vi "test Get Faultable Parameter.vi"() -> ()   [LabVIEW 2023, in "Scripting.lvclass"]
uses:
  Scripting.lvclass
  Scripting.lvclass/Scripting.ctl
  <vilib>/NI/NI VeriStand Encoding and Decoding/Encoding.ctl
  <vilib>/NI/NI VeriStand Encoding and Decoding/Encoding and Decoding.lvlib
  Shared/Parameter Definition.ctl
  Shared/Direction.ctl
  Shared/SDI.ctl
  Shared/Transfer Type.ctl
  Shared/Transfer Speed.ctl
  Scripting/AIM/AIM ARINC 429 Scripting.lvlib
  <vilib>/addons/_JKI Toolkits/VI Tester/TestCase.llb/TestCase.lvclass
  C:/Program Files/National Instruments/LabVIEW 2023/vi.lib/addons/_JKI Toolkits/VI Tester/TestCase.llb/TestCase.lvclass
  C:/repo/niveristand-aim-arinc429-custom-device/Source/Custom Device Support/Tests/Unit/Scripting/Scripting.lvclass
panel:
  out "TestCase out":refnum<class "Scripting.lvclass">
  in  "TestCase in":refnum<class "Scripting.lvclass">
  out "error out":errorcluster
  in  "error in":errorcluster
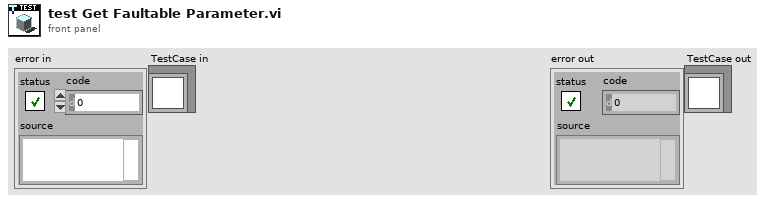
[diagram p1: front panel]
types:
  T1 = typedef "Transfer Speed.ctl" = enum16{"LO (12.5 kb/s)", "HI (100 kb/s)"}
  T2 = typedef "Transfer Type.ctl" = enum16{"Scheduled", "Acyclic", "Block", "Strobe"}
  T3 = typedef "Direction.ctl" = enum16{"Rx", "Tx"}
  T4 = typedef "SDI.ctl" = i32
  T5 = typedef "Parameter Definition.ctl" = cluster{"start index":i32, "size":i32, "encoding":T6, "signed":bool, "scale multiplier":dbl, "scale offset":dbl, "default value":dbl}
  T6 = typedef "Encoding and Decoding.lvlib/Encoding.ctl" = enum16{"BNR", "BCD", "Discrete"}
  T7 = typedef "Custom Device API.lvlib/Custom Device Item Ref.ctl" = u64
  T8 = typedef "Custom Device API.lvlib/Custom Device Channel.ctl" = cluster{"Type":T9, "Units":string, "Default Value":dbl, "Faultable":bool, "Scalable":bool}
  T9 = typedef "Custom Device API.lvlib/Custom Device Channel Type.ctl" = enum16{"Input", "Output"}
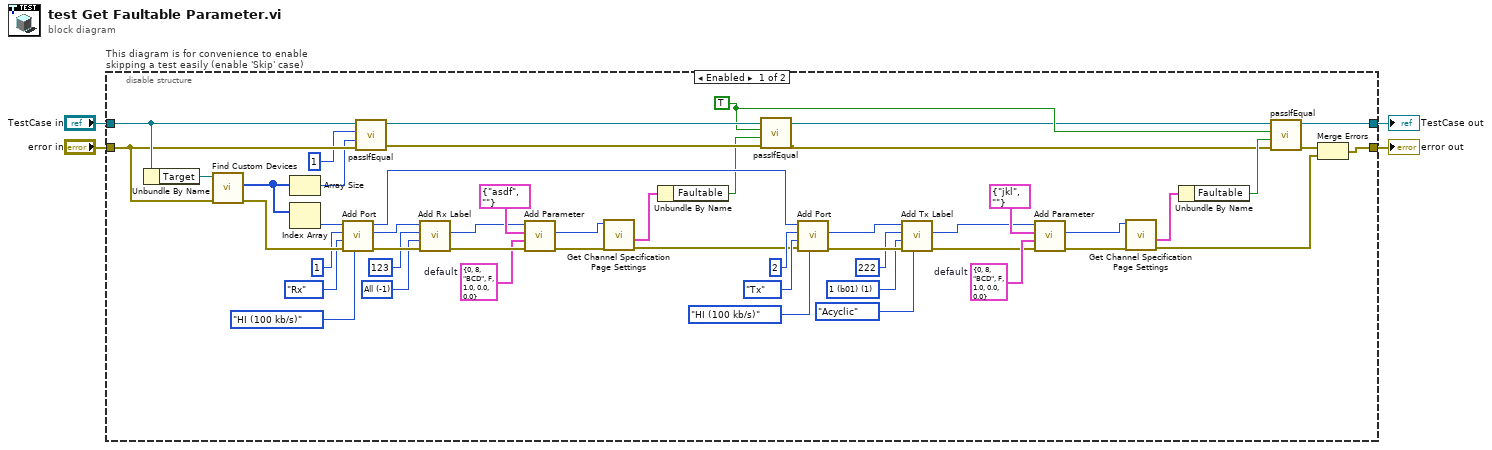
[diagram p0: block diagram]
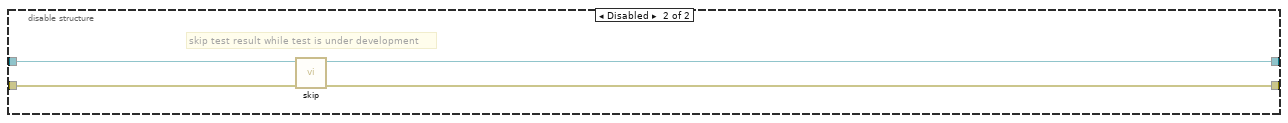
[diagram p2: hidden frame]
diagram:
  n1 = disable-structure "This diagram is for convenience to enable skipping a test easily (enable 'Skip' case)" shown="Enabled" {
    disable-tunnel: "TestCase in" -> [w53 w58]
    disable-tunnel: [w47 w56] -> w1
    disable-tunnel: [w49 w57] -> w3
    disable-tunnel: "error in" -> [w52 w55]
    frame Enabled {
      w8 = TRUE ("Faultable")
      w26 = T4 1 items=["All"=-1, "0 (b00)"=0, "1 (b01)"=1, "2 (b10)"=2, "3 (b11)"=3] ("SDI value")
      w32 = T5 {"start index"=0, "size"=8, "encoding"=enum."BCD", "signed"=FALSE, "scale multiplier"=1.0, "scale offset"=0.0, "default value"=0.0}  # default
      w33 = T5 {"start index"=0, "size"=8, "encoding"=enum."BCD", "signed"=FALSE, "scale multiplier"=1.0, "scale offset"=0.0, "default value"=0.0}  # default
      w36 = T4 -1 items=["All"=-1, "0 (b00)"=0, "1 (b01)"=1, "2 (b10)"=2, "3 (b11)"=3] ("SDI value")
      n2 = Unbundle By Name(w53) -> ("Target"=w54:refnum<k24>)
      n3 = call "Find Custom Devices.vi"("error in"=w52, "target"=w54) -> ("error out"=w44:errorcluster, "AIM ARINC 429 custom devices"=w46:T7[])  [unwired: 7 in, 1 out]
      n4 = Array Size(array=w46) -> (size(s)=w50:i32)
      n5 = Index Array(array=w46) -> (element=w45:T7)  [unwired: 1 in]
      n6 = call "Add Port.vi"("speed"=Transfer_Speed."HI (100 kb/s)", "error in"=w44, "direction"=Direction."Rx", "port number"=u16 1, "custom device ref"=w45) -> ("error out"=w38:errorcluster, "port"=w39:T7, "custom device ref out"=w25:T7)  [unwired: 4 in]
      n7 = call-dynamic "passIfEqual.vi"("error in (no error)"=w52, "y"=w50, "x"=1 ("size(s)"), "TestCase in"=w53) -> ("error out"=w17:errorcluster, "TestCase out"=w16:refnum<class "Scripting.lvclass">)  [unwired: 6 in]
      n8 = call "Add Rx Label.vi"("error in"=w38, "SDI value"=w36, "label value"=u32 123, "port ref"=w39) -> ("error out"=w34:errorcluster, "label"=w23:T7)  [unwired: 5 in, 1 out]
      n9 = call "Add Parameter.vi"("error in"=w34, "parameter encoding"=w33, "parameter definition"=cluster{"name":string, "unit":string} {"name"="asdf", "unit"=""}, "label ref"=w23) -> ("error out"=w14:errorcluster, "parameter"=w19:T7)  [unwired: 5 in, 1 out]
      n10 = call "Get Channel Specification Page Settings.vi"("error in"=w14, "parameter ref"=w19) -> ("error out"=w13:errorcluster, "Channel"=w18:T8)  [unwired: 6 in, 2 out]
      n11 = Unbundle By Name(w18) -> ("Faultable"=w15:bool)
      n12 = call-dynamic "passIfEqual.vi"("error in (no error)"=w17, "y"=w15, "x"=w8, "TestCase in"=w16) -> ("error out"=w6:errorcluster, "TestCase out"=w7:refnum<class "Scripting.lvclass">)  [unwired: 6 in]
      n13 = call "Add Port.vi"("speed"=Transfer_Speed."HI (100 kb/s)", "error in"=w13, "direction"=Direction."Tx", "port number"=u16 2, "custom device ref"=w25) -> ("error out"=w30:errorcluster, "port"=w29:T7)  [unwired: 4 in, 1 out]
      n14 = call "Add Tx Label.vi"("transfer type"=Transfer_Type."Acyclic", "error in"=w30, "SDI value"=w26, "label value"=u32 222, "port ref"=w29) -> ("error out"=w28:errorcluster, "label"=w22:T7)  [unwired: 4 in, 1 out]
      n15 = call "Add Parameter.vi"("error in"=w28, "parameter encoding"=w32, "parameter definition"=cluster{"name":string, "unit":string} {"name"="jkl", "unit"=""}, "label ref"=w22) -> ("error out"=w11:errorcluster, "parameter"=w10:T7)  [unwired: 5 in, 1 out]
      n16 = call "Get Channel Specification Page Settings.vi"("error in"=w11, "parameter ref"=w10) -> ("error out"=w5:errorcluster, "Channel"=w12:T8)  [unwired: 6 in, 2 out]
      n17 = Unbundle By Name(w12) -> ("Faultable"=w9:bool)
      n18 = call-dynamic "passIfEqual.vi"("error in (no error)"=w6, "y"=w9, "x"=w8, "TestCase in"=w7) -> ("error out"=w48:errorcluster, "TestCase out"=w47:refnum<class "Scripting.lvclass">)  [unwired: 6 in]
      n19 = Merge Errors(w48, w5) -> (w49:errorcluster)
    }
    frame Disabled {
      # "skip test result while test is under development"
      n20 = call <vilib>:"skip.vi"("error in (no error)"=w55, "TestCase in"=w58) -> ("error out"=w57:errorcluster, "TestCase out"=w56:refnum<class "Scripting.lvclass">)  [unwired: 8 in]
    }
  }
  "error out" <- w3
  "TestCase out" <- w1
